vi "Chassis Initialize.vi"(8 "error in (no error)":errorcluster, 9 "Reset (True)":bool=TRUE, 10 "ID Query (True)":bool=TRUE, 11 "Chassis VISA resource name":refnum<visa-resource-name>) -> (0 "error out":errorcluster, 3 "Chassis VISA resource name out":refnum<visa-resource-name>)   [LabVIEW 2018, in "Agilent U2722.lvlib"]
doc: "Establishes communication with the chassis and optionally performs an chassis identification query and/or an chassis reset. It also places the chassis in a default state needed for other instrument driver operations. Therefore, call this VI before calling other chassis driver VIs for this instrument. Generally, you need to call the Chassis Initialize VI only once at the beginning of an application relative to chassis."
uses:
  <instrlib>/Agilent U2722/Agilent U2722.lvlib
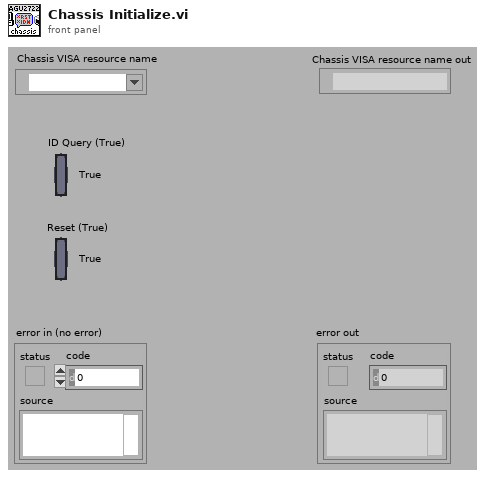
[diagram p1: front panel]
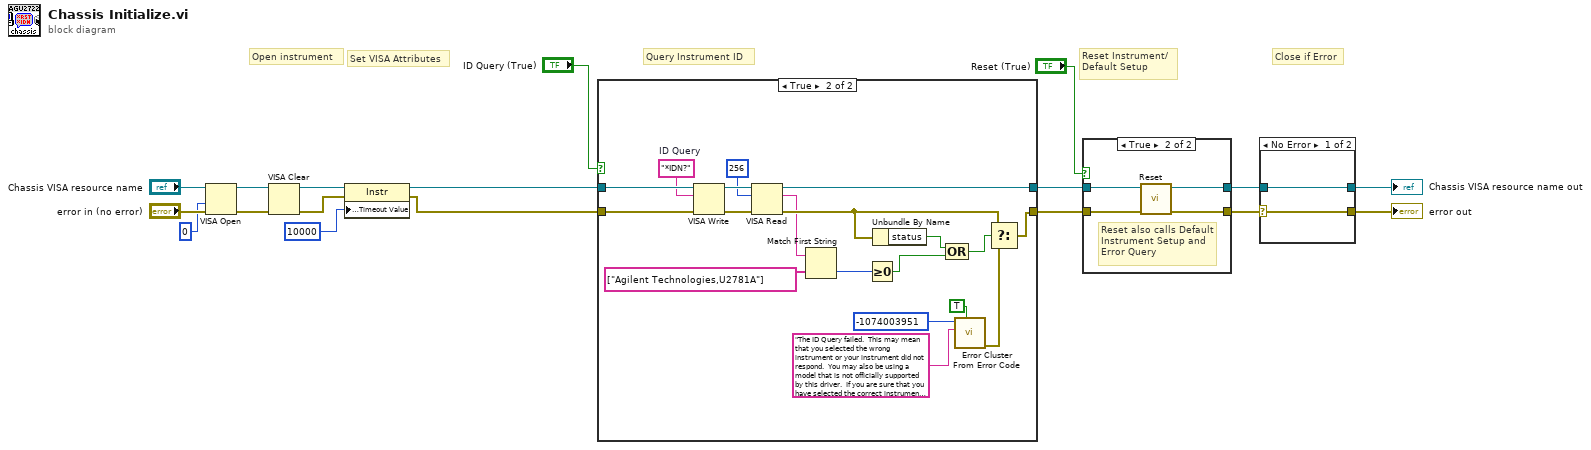
[diagram p0: block diagram]
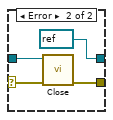
[diagram p2: hidden frame]
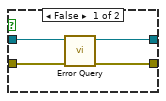
[diagram p3: hidden frame]
diagram:
  # "Set VISA Attributes"
  # "Close if Error"
  # "Query Instrument ID"
  # "Reset Instrument/\nDefault Setup"
  # "Open instrument"
  n1 = VISA Open(access mode=u32 0, error in (no error)="error in (no error)", VISA resource name="Chassis VISA resource name") -> (VISA resource name=w10:refnum<visa-resource-name>, error out=w9:errorcluster)  [unwired: 2 in]
  n2 = VISA Clear(VISA resource name=w10, error in (no error)=w9) -> (VISA resource name out=w8:refnum<visa-resource-name>, error out=w7:errorcluster)
  n3 = property class="Instr"(reference=w8, error in=w7, "General Settings:Timeout Value"=u32 10000) -> (reference out=w2:refnum<visa-resource-name>, error out=w1:errorcluster)
  n4 = case shown="True" "ID Query (True)" {
    tunnel: [w19 w39] -> w17
    tunnel: [w20 w36] -> w18
    tunnel: w2 -> [w20 w37]
    tunnel: w1 -> [w19 w38]
    frame False {
    }
    frame True {
      w32 = "*IDN?"  # ID Query
      n5 = VISA Write(VISA resource name=w37, write buffer=w32, error in (no error)=w38) -> (VISA resource name out=w35:refnum<visa-resource-name>, error out=w34:errorcluster)  [unwired: 1 out]
      n6 = VISA Read(VISA resource name=w35, byte count=u32 256, error in (no error)=w34) -> (VISA resource name out=w36:refnum<visa-resource-name>, read buffer=w22:string, error out=w27:errorcluster)  [unwired: 1 out]
      n7 = Match First String(2:string[] ["Agilent Technologies,U2781A"] ("string array"), 3:w22) -> (0:w23:i32)  [unwired: 1 out]
      n8 = Greater Or Equal To 0?(x=w23) -> (x >= 0?=w25:bool)
      n9 = Unbundle By Name(w27) -> ("status"=w26:bool)
      n10 = Compound Arithmetic op=OR(w26, w25) -> (w24:bool)
      n11 = call <vilib>:"Error Cluster From Error Code.vi"("show call chain? (False)"=TRUE, "error message (\"\")"="The ID Query failed.  This may mean that you selected the wrong instrument or your instrument did not respond.  You may also be using a model that is not officially supported by this driver.  If you are sure that you have selected the correct instrument and it is responding, try disabling the ID Query." ("Source (VI Name)"), "error code (0)"=-1074003951 ("Code")) -> ("error out"=w31:errorcluster)  [unwired: 6 in]
      n12 = Select(t=w27, s=w24, f=w31) -> (s? t:f=w39:errorcluster)
    }
  }
  n13 = case shown="True" "Reset (True)" {
    tunnel: w17 -> [w40 w44]
    tunnel: [w42 w47] -> w3
    tunnel: w18 -> [w41 w45]
    tunnel: [w43 w46] -> w4
    frame False {
      n14 = call <instrlib>:"Error Query.vi"("error in (no error)"=w40, "VISA resource name"=w41) -> ("error out"=w42:errorcluster, "VISA resource name out"=w43:refnum<visa-resource-name>)  [unwired: 6 in, 2 out]
    }
    frame True {
      # "Reset also calls Default Instrument Setup and Error Query"
      n15 = call <instrlib>:"Reset.vi"("error in (no error)"=w44, "VISA resource name"=w45) -> ("error out"=w47:errorcluster, "VISA resource name out"=w46:refnum<visa-resource-name>)  [unwired: 8 in]
    }
  }
  n16 = case shown="No Error" w3 {
    selector: w3 -> [w48 w51]
    tunnel: w4 -> [w49 w52]
    tunnel: [w49 refnum<visa-resource-name> refnum ("VISA resource name out")] -> w6
    tunnel: [w48 w53] -> w5
    frame No Error {
    }
    frame Error {
      n17 = call <instrlib>:"Close.vi"("error in (no error)"=w51, "VISA resource name"=w52) -> ("error out"=w53:errorcluster)  [unwired: 9 in]
    }
  }
  "Chassis VISA resource name out" <- w6
  "error out" <- w5
